vi "PXIe-7903 Aurora Example Host (2-port).vi"() -> ()   [LabVIEW 2023]
uses:
  <vilib>/userDefined/High Color/nirio_resource_hc.ctl
  <instrlib>/_niInstr/Aurora64b66b/v1/Host/Interface/Public/TypeDefs/Differential Voltage Swing (mV).ctl
  <instrlib>/_niInstr/Aurora64b66b/v1/Host/Interface/Public/TypeDefs/Tx Emphasis (dB).ctl
  <instrlib>/_niInstr/Aurora64b66b/v1/Shared/Basic/Aurora Config.ctl
  <instrlib>/_niInstr/Aurora64b66b/v1/Shared/Basic/GT Type.ctl
  <instrlib>/_niInstr/Aurora64b66b/v1/Shared/Basic/Endianness.ctl
  <instrlib>/_niInstr/Aurora64b66b/v1/Host/Interface/Public/TypeDefs/Counters.ctl
  <instrlib>/_niInstr/Aurora64b66b/v1/Host/Interface/Public/TypeDefs/Link Status.ctl
  <instrlib>/_niInstr/FIFO Register Bus/v1/Host/niInstr FIFO Register Bus v1 Host.lvclass
  <instrlib>/_niInstr/Instruction Framework/v1/Host/Subsystem Map/Private/Lookup Single Context.vi
  <vilib>/Utility/error.llb/Error Cluster From Error Code.vi
  <vilib>/rvi/errors/niLvFpgaAdjustHostInterfaceError.vi
  <vilib>/ErrorRing/Error Ring.xnode
  <vilib>/rvi/interface/nirviReadWriteControl/nirviReadWriteControl.xnode
  <vilib>/rvi/interface/nirviCloseFPGA/nirviCloseFPGA.xnode
  <instrlib>/_niInstr/Aurora64b66b/v1/Host/Interface/Aurora64b66b.lvclass
  <vilib>/rvi/interface/Simulation/niFpgaSimulationCallBeginRW.vi
  <instrlib>/_niInstr/Instruction Framework/v1/Host/Subsystem Map/niInstr Subsystem Map v1 Host.lvclass
  NiFpgaLv.dll
  PXIe-7903 Aurora Example Host.lvlib
  C:/Program Files/NI/LVAddons/niidl/1/instr.lib/_niInstr/Instruction Framework/v1/Host/Instruction Target/niInstr Instruction Target v1 Host.lvclass
  C:/Program Files/NI/LVAddons/niidl/1/instr.lib/_niInstr/FIFO Register Bus/v1/Host/niInstr FIFO Register Bus v1 Host.lvclass
  <vilib>/FPGAPlugInAG/Dynamic/niLvFpga_Close_Dynamic.vi
  <instrlib>/_niInstr/Aurora64b66b/v1/Shared/niInstr Aurora64b66b v1 Shared.lvlib
panel:
  out "tx fifo overflow":bool[](array[boolean])
  out "link status":T1[](array[typedef])
  out "counters":T2[](array[typedef])
  out "rx fifo overflow":bool[](array[boolean])
  out "rx throughput":dbl[](array[numeric])
  out "tx throughput":dbl[](array[numeric])
  out "mismatch count":u64[](array[numeric])
  in  "frame size":u16
  in  "rx throttle":u16=65535
  out "port config":T3[](array[typedef]) {"line rate" format="%.6p"; "ref clk frequency" format="%.6p"}
  in  "second aurora instance":u8=2
  in  "first aurora instance":u8
  out "error out":errorcluster
  in  "reset counters":bool
  in  "stop":bool
  in  "pre-emphasis (dB)":T6
  in  "post-emphasis (dB)":T6
  in  "differential swing (mV)":T7=enum."695"
  in  "device":T8
  in  "bitfile":path
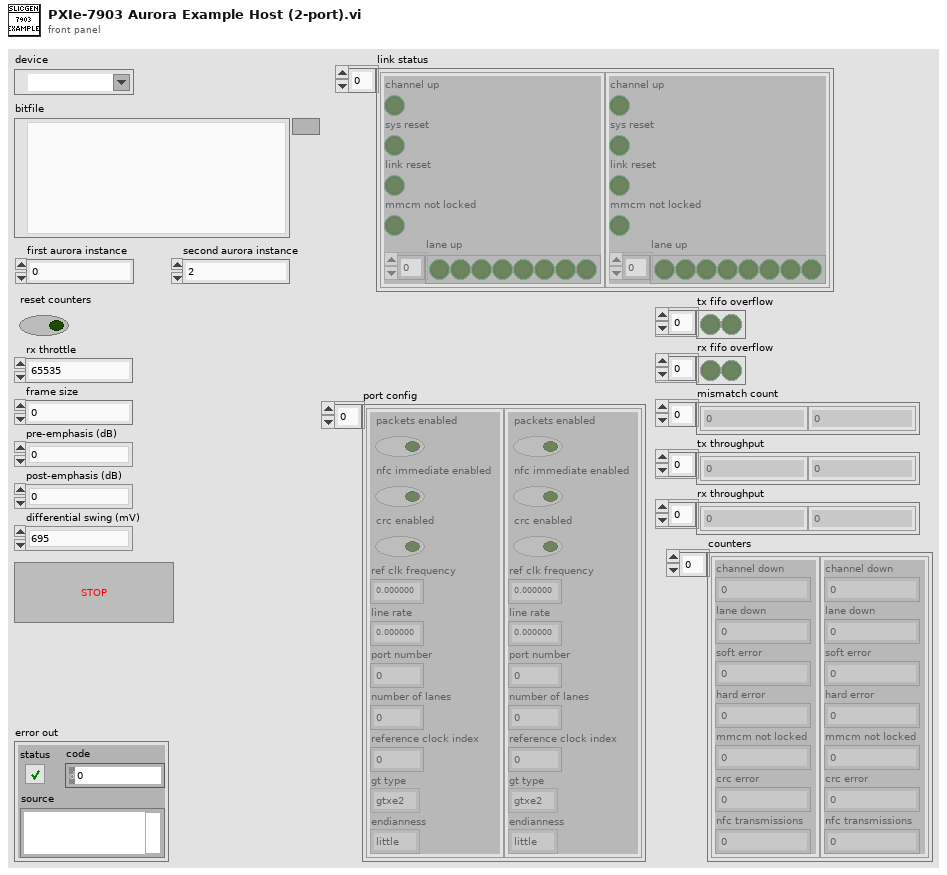
[diagram p1: front panel]
types:
  T1 = typedef "niInstr Aurora64b66b v1 Host.lvlib/Aurora64b66b.lvclass/Link Status.ctl" = cluster{"channel up":bool, "sys reset":bool, "link reset":bool, "mmcm not locked":bool, "lane up":bool[]}
  T2 = typedef "niInstr Aurora64b66b v1 Host.lvlib/Aurora64b66b.lvclass/Counters.ctl" = cluster{"channel down":u32, "lane down":u32, "soft error":u32, "hard error":u32, "mmcm not locked":u32, "crc error":u32, "nfc transmissions":u64}
  T3 = typedef "niInstr Aurora64b66b v1 Shared.lvlib/Aurora Config.ctl" = cluster{"packets enabled":bool, "nfc immediate enabled":bool, "crc enabled":bool, "ref clk frequency":u64, "line rate":u64, "port number":u8, "number of lanes":u8, "reference clock index":u8, "gt type":T4, "endianness":T5}
  T4 = typedef "niInstr Aurora64b66b v1 Shared.lvlib/GT Type.ctl" = enum16{"gtxe2", "gthe2", "gthe3", "gtye4"}
  T5 = typedef "niInstr Aurora64b66b v1 Shared.lvlib/Endianness.ctl" = enum16{"little", "big"}
  T6 = typedef "niInstr Aurora64b66b v1 Host.lvlib/Aurora64b66b.lvclass/Tx Emphasis (dB).ctl" = enum16{"0", "0.22", "0.45", "0.68", "0.92", "1.16", "1.41", "1.67", "1.94", "2.21", "2.50", "2.79", "3.10", "3.41", "3.74", "4.08", "4.44", "4.81", "5.19", "5.60", "6.02", "6.47", "6.94", "7.43", "7.96", "8.52", "9.12", "9.76", "10.46", "11.21", "12.04", "12.96"}
  T7 = typedef "niInstr Aurora64b66b v1 Host.lvlib/Aurora64b66b.lvclass/Differential Voltage Swing (mV).ctl" = enum16{"191", "223", "254", "286", "315", "347", "378", "408", "439", "470", "499", "529", "556", "585", "613", "640", "669", "695", "720", "744", "766", "788", "809", "828", "846", "863", "878", "892", "903", "914", "924", "933"}
  T8 = typedef "nirio_resource_hc.ctl" = tag
  T9 = enum16{"<invalid>", "<menus>", "<vilib>", "<userlib>", "<instrlib>", "<helpdir>", "<libdir>", "<osdatadir>", "<nishared>", "<instcachedir>", "<resource>", "<extravilib>"}
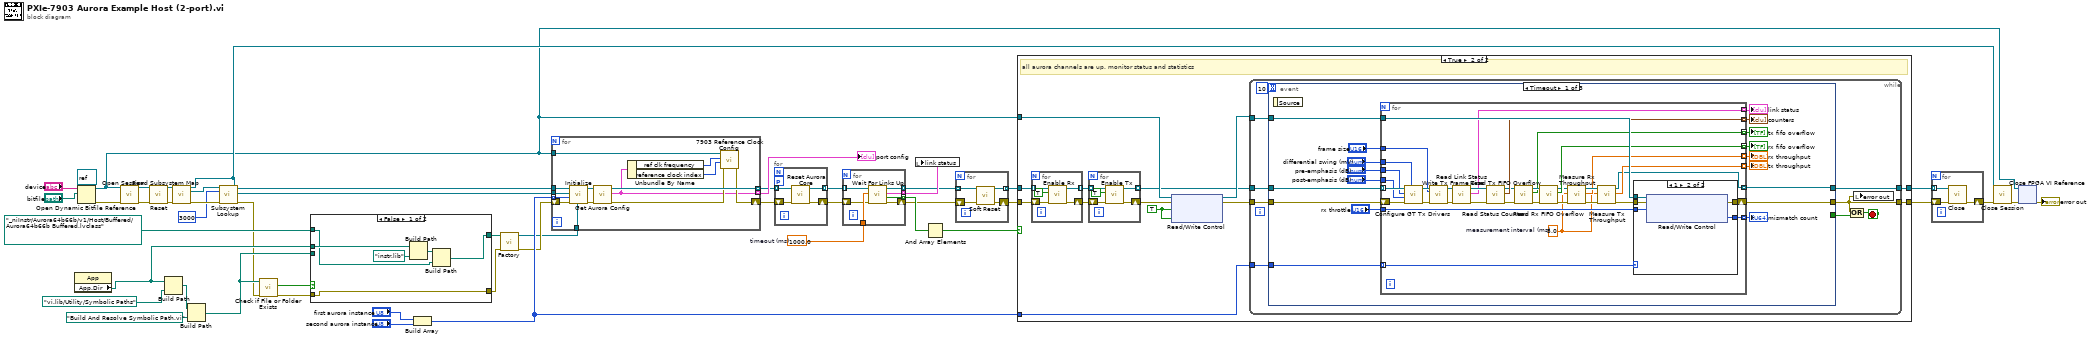
[diagram p0: block diagram]
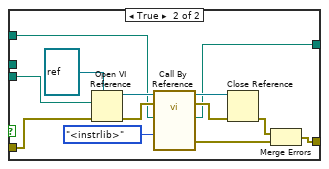
[diagram p2: hidden frame]
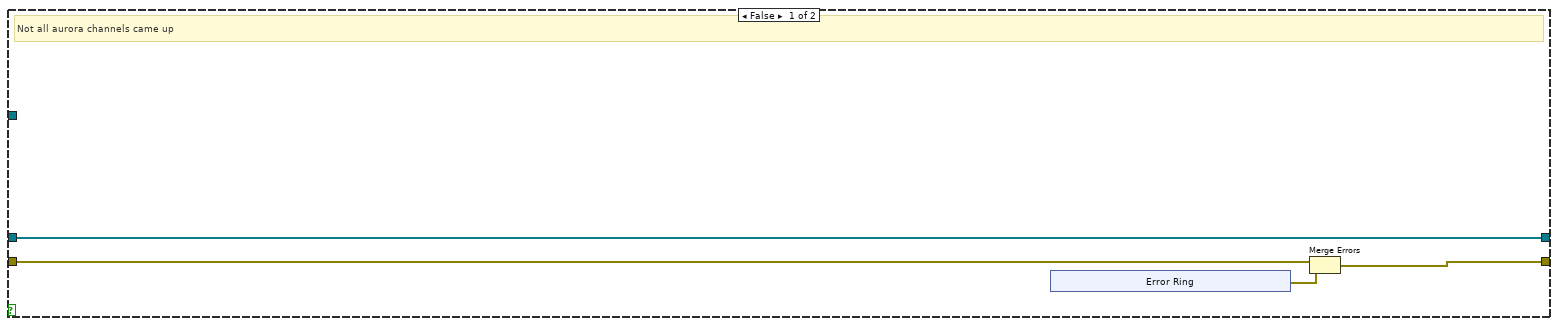
[diagram p3: hidden frame]
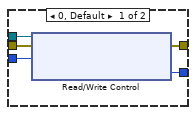
[diagram p4: hidden frame]
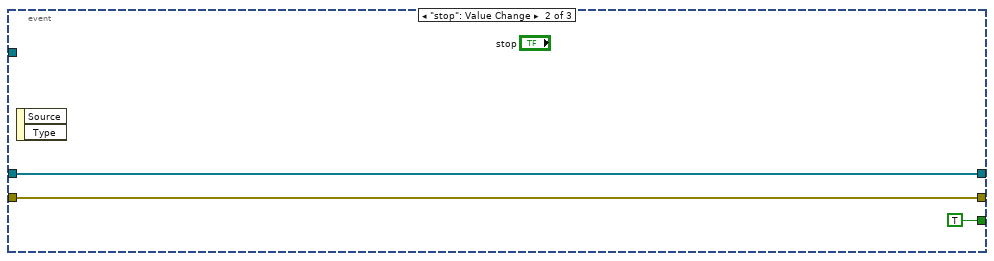
[diagram p5: hidden frame]
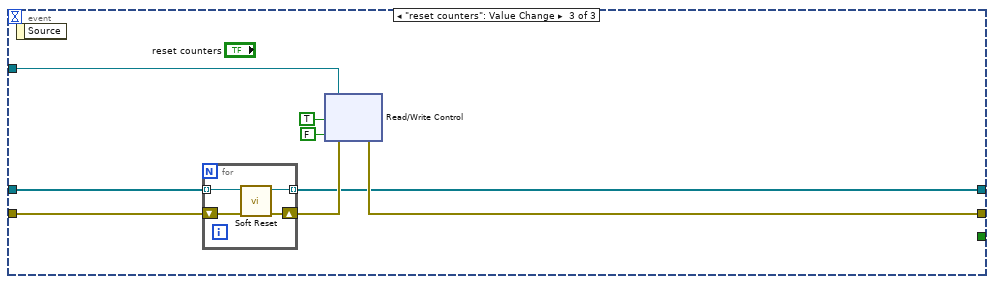
[diagram p6: hidden frame]
diagram:
  w43 = 1000.0  # timeout (ms)
  n1 = property class="App"() -> ("App.Dir"=w10:path)  [unwired: 2 in, 2 out]
  n2 = Open Dynamic Bitfile Reference(0:"device", 1:"bitfile", 4:refnum<k20> refnum ("Type")) -> (5:w28:refnum<k20>, 8:w27:errorcluster)  [unwired: 2 in]
  n3 = call <instrlib>:"Open Session.vi"("fpga ref"=w28, "error in"=w27) -> ("session out"=w31:refnum<class "niInstr FIFO Register Bus v1 Host.lvclass">, "error out"=w30:errorcluster)  [unwired: 12 in]
  n4 = call-dynamic "Reset.vi"("session in"=w31, "error in"=w30) -> ("session out"=w32:refnum<class "niInstr FIFO Register Bus v1 Host.lvclass">, "error out"=w29:errorcluster)  [unwired: 12 in]
  n5 = Build Path(base path=w10, name or relative path=path "vi.lib/Utility/Symbolic Paths" ("path")) -> (appended path=w12:path)
  n6 = call <instrlib>:"Read Subsystem Map.vi"("instruction target in"=w32, "error in"=w29) -> ("instruction target out"=w42:refnum<class "niInstr FIFO Register Bus v1 Host.lvclass">, "subsystem map"=w45:refnum<class "niInstr Subsystem Map v1 Host.lvclass">, "error out"=w44:errorcluster)  [unwired: 11 in]
  n7 = Build Path(base path=w12, name or relative path=path "Build And Resolve Symbolic Path.vi") -> (appended path=w11:path)
  n8 = call-poly <instrlib>:"Subsystem Lookup.vi"("subsystem map in"=w45, "UID"=u16 3000, "error in"=w44) -> ("context"=w41:refnum<class "niInstr Instruction Framework Context v1 Host.lvclass">, "error out"=w6:errorcluster)  [unwired: 9 in, 2 out]
  n9 = call <vilib>:"Check if File or Folder Exists.vi"("error in (no error)"=w6, "path"=w11) -> ("error out"=w14:errorcluster, "file or folder exists?"=w15:bool)  [unwired: 7 in, 1 out]
  n10 = case shown="False" w15 {
    tunnel: path "_niInstr/Aurora64b66b/v1/Host/Buffered/Aurora64b66b Buffered.lvclass" ("name or relative path") -> [w50 w64]
    tunnel: w11 -> [_ w58]
    tunnel: [w54 w55] -> w5
    tunnel: w14 -> [w54 w60]
    tunnel: [w49 w59] -> w8
    tunnel: w10 -> [w53 _]
    frame False {
      n11 = Build Path(base path=w53, name or relative path=path "instr.lib") -> (appended path=w52:path)
      n12 = Build Path(base path=w52, name or relative path=w50) -> (appended path=w49:path)
    }
    frame True {
      n13 = Open VI Reference(type specifier VI Refnum (for type only)=refnum<vi> refnum, vi path=w58, error in (no error)=w60) -> (vi reference=w66:refnum<vi>, error out=w65:errorcluster)  [unwired: 3 in]
      n14 = call-by-ref "?"(reference=w66, error in=w65, "symbolic path id (<vilib>)"=T9."<instrlib>", "relative path"=w64) -> (reference out=w61:refnum<vi>, error out=w62:errorcluster, 0:"error out"=w56:errorcluster, "resolved path"=w59:path)  [unwired: 7 in, 1 out]
      n15 = Close Reference(reference=w61, error in (no error)=w62) -> (error out=w57:errorcluster)
      n16 = Merge Errors(w57, w56) -> (w55:errorcluster)
    }
  }
  n17 = Build Array("first aurora instance", "second aurora instance") -> (w34:u8[])
  n18 = call <instrlib>:"Factory.vi"("error in"=w5, "class path"=w8) -> ("error out"=w26:errorcluster, "aurora64b66b"=w25:refnum<class "Aurora64b66b.lvclass">)  [unwired: 8 in]
  n19 = for {
    tunnel: w42 -> [w76]
    tunnel: w41 -> [w75]
    shift-right: [w71] -> w22
    shift-left: w26 -> [w81]
    tunnel: w34 -> [w74] mode=indexing
    tunnel: w25 -> [w79]
    tunnel: [w80] -> w21 mode=indexing
    tunnel: [w70] -> w35 mode=indexing
    tunnel: w28 -> [w73]
    n20 = call-dynamic "Initialize.vi"("select session"=w79, "error in"=w81, "instance (0)"=w74, "parent context (root)"=w75, "register bus"=w76) -> ("error out"=w78:errorcluster, "aurora64b66b"=w77:refnum<class "Aurora64b66b.lvclass">)  [unwired: 5 in]
    n21 = call-dynamic "Get Aurora Config.vi"("error in"=w78, "aurora64b66b in"=w77) -> ("error out"=w72:errorcluster, "aurora config"=w70:T3, "aurora64b66b out"=w80:refnum<class "Aurora64b66b.lvclass">)  [unwired: 7 in]
    n22 = Unbundle By Name(w70) -> ("ref clk frequency"=w69:u64, "reference clock index"=w68:u8)
    n23 = call "7903 Reference Clock Config.vi"("error in"=w72, "reference clock index"=w68, "ref clk frequency"=w69, "fpga interface in"=w73) -> ("error out"=w71:errorcluster)  [unwired: 6 in, 1 out]
  }
  "port config" <- w35
  n24 = for {
    shift-right: [w84] -> w19
    shift-left: w22 -> [w85]
    tunnel: w21 -> [w83] mode=indexing
    tunnel: [w82] -> w20 mode=indexing
    workers-P: _ -> [_]
    n25 = call <instrlib>:"Reset Aurora Core.vi"("error in"=w85, "aurora64b66b in"=w83) -> ("error out"=w84:errorcluster, "aurora64b66b out"=w82:refnum<class "Aurora64b66b.lvclass">)  [unwired: 8 in]
  }
  n26 = for {
    tunnel: w43 -> [w91]
    tunnel: [w90] -> w24 mode=indexing
    tunnel: [w89] -> w4 mode=indexing
    tunnel: [w88] -> w33 mode=indexing
    shift-right: [w92] -> w2
    shift-left: w19 -> [w87]
    tunnel: w20 -> [w86] mode=indexing
    n27 = call <instrlib>:"Wait For Links Up.vi"("error in"=w87, "timeout (ms)"=w91, "aurora64b66b in"=w86) -> ("error out"=w92:errorcluster, "channel up"=w90:bool, "link status"=w88:T1, "aurora64b66 out"=w89:refnum<class "Aurora64b66b.lvclass">)  [unwired: 5 in]
  }
  n28 = local write "link status"(w33) -> ()
  n29 = And Array Elements(Boolean array=w24) -> (logical AND=w23:bool)
  n30 = for {
    tunnel: w4 -> [w96] mode=indexing
    tunnel: [w95] -> w3 mode=indexing
    shift-right: [w94] -> w1
    shift-left: w2 -> [w93]
    n31 = call-dynamic "Soft Reset.vi"("error in"=w93, "aurora64b66b in"=w96) -> ("error out"=w94:errorcluster, "aurora64b66b out"=w95:refnum<class "Aurora64b66b.lvclass">)  [unwired: 8 in]
  }
  n32 = case shown="True" w23 {
    tunnel: [w100 w118] -> w17
    tunnel: w3 -> [w97 w113]
    tunnel: w1 -> [w99 w114]
    tunnel: w28 -> [_ w111]
    tunnel: w34 -> [_ w117]
    tunnel: [w97 w112] -> w18
    frame False {
      # "Not all aurora channels came up"
      n33 = xnode "Error Ring"() -> ("error out"=w98:errorcluster)
      n34 = Merge Errors(w99, w98) -> (w100:errorcluster)
    }
    frame True {
      w106 = TRUE ("port 0 enable")
      # "all aurora channels are up. monitor status and statistics"
      n35 = for {
        tunnel: w113 -> [w123] mode=indexing
        tunnel: [w122] -> w116 mode=indexing
        shift-right: [w121] -> w115
        shift-left: w114 -> [w120]
        n36 = call-dynamic "Enable Rx.vi"("error in"=w120, "enable"=TRUE, "aurora64b66b in"=w123) -> ("error out"=w121:errorcluster, "aurora64b66b out"=w122:refnum<class "Aurora64b66b.lvclass">)  [unwired: 7 in]
      }
      n37 = for {
        tunnel: w116 -> [w128] mode=indexing
        tunnel: [w127] -> w107 mode=indexing
        shift-right: [w126] -> w109
        shift-left: w115 -> [w125]
        n38 = call-dynamic "Enable Tx.vi"("error in"=w125, "enable"=TRUE, "aurora64b66b in"=w128) -> ("error out"=w126:errorcluster, "aurora64b66b out"=w127:refnum<class "Aurora64b66b.lvclass">)  [unwired: 7 in]
      }
      n39 = xnode "Read/Write Control"("FPGA VI Reference In"=w111, "error in"=w109, "port 0 enable"=w106, "port 1 enable"=w106) -> ("FPGA VI Reference Out"=w110:refnum<k20>, "error out"=w108:errorcluster)
      n40 = while {
        tunnel: [w137] -> w118
        tunnel: w107 -> [w133]
        tunnel: w108 -> [w134]
        tunnel: w110 -> [w131]
        tunnel: w117 -> [w130]
        tunnel: [w129] -> w112
        stop <- w135 stop-if-true
        n41 = event shown="[0] Timeout" {
          selector: _ -> [_ _ _]
          dyn-events: _ -> [_ _ _]
          timeout: 10 -> [_ _ _]
          tunnel: [w139 w200 w204] -> w137
          tunnel: [_ TRUE ("stop") _] -> w136
          tunnel: w134 -> [w154 w200 w210]
          tunnel: w133 -> [w155 w201 w209]
          tunnel: w131 -> [w150 _ w208]
          tunnel: w130 -> [w149 _ _]
          tunnel: [w138 w201 w203] -> w129
          event Timeout {
            n42 = event-data() -> ()  [unwired: 1 in, 1 out]
            n43 = for {
              tunnel: w155 -> [w189] mode=indexing
              tunnel: "pre-emphasis (dB)" -> [w187]
              tunnel: "post-emphasis (dB)" -> [w186]
              tunnel: "differential swing (mV)" -> [w185]
              tunnel: w150 -> [w184]
              tunnel: [w180] -> w143 mode=indexing
              tunnel: [w179] -> w145 mode=indexing
              tunnel: [w177] -> w144 mode=indexing
              shift-right: [w178] -> w139
              shift-left: w154 -> [w188]
              tunnel: w149 -> [w176] mode=indexing
              tunnel: [w175] -> w146 mode=indexing
              tunnel: "rx throttle" -> [w174]
              tunnel: "frame size" -> [w156]
              tunnel: [w169] -> w142 mode=indexing
              tunnel: [w163] -> w141 mode=indexing
              tunnel: [w162] -> w140 mode=indexing
              tunnel: [w160] -> w138 mode=indexing
              w161 = 5.0  # measurement interval (ms)
              n44 = call-dynamic "Configure GT Tx Drivers.vi"("differential swing (mv)"=w185, "error in"=w188, "post-emphasis (dB)"=w186, "pre-emphasis (dB)"=w187, "aurora64b66b in"=w189) -> ("error out"=w181:errorcluster, "aurora64b66b out"=w158:refnum<class "Aurora64b66b.lvclass">)  [unwired: 5 in]
              n45 = call-dynamic "Write Tx Frame Size.vi"("error in"=w181, "tx frame size"=w156, "aurora64b66b in"=w158) -> ("error out"=w159:errorcluster, "aurora64b66b out"=w157:refnum<class "Aurora64b66b.lvclass">)  [unwired: 7 in]
              n46 = call-dynamic "Read Link Status.vi"("error in"=w159, "aurora64b66b in"=w157) -> ("error out"=w182:errorcluster, "link status"=w180:T1, "aurora64b66b out"=w183:refnum<class "Aurora64b66b.lvclass">)  [unwired: 7 in]
              n47 = call-dynamic "Read Status Counters.vi"("error in"=w182, "aurora64b66b in"=w183) -> ("error out"=w171:errorcluster, "counters"=w177:T2, "aurora64b66b out"=w173:refnum<class "Aurora64b66b.lvclass">)  [unwired: 7 in]
              n48 = call-dynamic "Read Tx FIFO Overflow.vi"("error in"=w171, "aurora64b66b in"=w173) -> ("error out"=w170:errorcluster, "tx fifo overflow"=w169:bool, "aurora64b66b out"=w172:refnum<class "Aurora64b66b.lvclass">)  [unwired: 7 in]
              n49 = call-dynamic "Read Rx FIFO Overflow.vi"("error in"=w170, "aurora64b66b in"=w172) -> ("error out"=w166:errorcluster, "rx fifo overflow"=w179:bool, "aurora64b66b out"=w168:refnum<class "Aurora64b66b.lvclass">)  [unwired: 7 in]
              n50 = call-dynamic "Measure Rx Throughput.vi"("error in"=w166, "measurement interval (ms)"=w161, "aurora64b66b in"=w168) -> ("error out"=w165:errorcluster, "throughput (bps)"=w163:dbl, "aurora64b66b out"=w167:refnum<class "Aurora64b66b.lvclass">)  [unwired: 6 in]
              n51 = call-dynamic "Measure Tx Throughput.vi"("error in"=w165, "measurement interval (ms)"=w161, "aurora64b66b in"=w167) -> ("error out"=w164:errorcluster, "throughput (bps)"=w162:dbl, "aurora64b66b out"=w160:refnum<class "Aurora64b66b.lvclass">)  [unwired: 6 in]
              n52 = case shown="1" w176 {
                tunnel: w184 -> [w194 w199]
                tunnel: w164 -> [w193 w198]
                tunnel: [w192 w197] -> w178
                tunnel: [w191 w196] -> w175
                tunnel: w174 -> [w190 w195]
                frame 0, Default {
                  n53 = xnode "Read/Write Control"("FPGA VI Reference In"=w194, "error in"=w193, "port 0 rx throttle"=w190) -> ("error out"=w192:errorcluster, "port 0 mismatch count"=w191:u64)  [unwired: 1 out]
                }
                frame 1 {
                  n54 = xnode "Read/Write Control"("FPGA VI Reference In"=w199, "error in"=w198, "port 1 rx throttle"=w195) -> ("error out"=w197:errorcluster, "port 1 mismatch count"=w196:u64)  [unwired: 1 out]
                }
              }
            }
            "mismatch count" <- w146
            "tx throughput" <- w140
            "rx throughput" <- w141
            "rx fifo overflow" <- w145
            "counters" <- w144
            "link status" <- w143
            "tx fifo overflow" <- w142
          }
          event "stop": Value Change {
            n55 = event-data() -> ()  [unwired: 1 in, 2 out]
          }
          event "reset counters": Value Change {
            n56 = event-data() -> ()  [unwired: 1 in, 1 out]
            n57 = for {
              tunnel: w209 -> [w213] mode=indexing
              shift-right: [w212] -> w207
              shift-left: w210 -> [w214]
              tunnel: [w211] -> w203 mode=indexing
              n58 = call-dynamic "Soft Reset.vi"("error in"=w214, "aurora64b66b in"=w213) -> ("error out"=w212:errorcluster, "aurora64b66b out"=w211:refnum<class "Aurora64b66b.lvclass">)  [unwired: 8 in]
            }
            n59 = xnode "Read/Write Control"("FPGA VI Reference In"=w208, "error in"=w207, "tb reset"=TRUE ("reset mismatch count"), "tb reset"=FALSE) -> ("error out"=w204:errorcluster)  [unwired: 1 out]
          }
        }
        n60 = Compound Arithmetic op=OR(w137, w136) -> (w135:bool)
        n61 = local write "error out"(w137) -> ()
      }
    }
  }
  n62 = for {
    tunnel: w18 -> [w217] mode=indexing
    shift-right: [w216] -> w16
    shift-left: w17 -> [w215]
    n63 = call-dynamic "Close.vi"("error in"=w215, "aurora64b66b in"=w217) -> ("error out"=w216:errorcluster)  [unwired: 9 in]
  }
  n64 = call-dynamic "Close Session.vi"("session in"=w42, "error in"=w16) -> ("error out"=w40:errorcluster)  [unwired: 13 in]
  n65 = xnode "Close FPGA VI Reference"("FPGA VI Reference In"=w28, "error in"=w40) -> ("error out"=→"error out":errorcluster)
